vi "GeoData.vi"() -> ()   [LabVIEW 2017] (continued)
County\tH1\n39365\t28123\tUnion\tMS\tScott County\tH1\n39098\t28123\tLudlow\tMS\tScott County\tH1\n39117\t28123\tMorton\tMS\tScott County\tH1\n39152\t28123\tPulaski\tMS\tScott County\tH1\n39359\t28123\tSebastopol\tMS\tScott County\tH1\n39092\t28123\tLake\tMS\tScott County\tH1\n39145\t28123\tPelahatchie\tMS\tScott County\tH1\n39189\t28123\tWalnut grove\tMS\tScott County\tH1\n39074\t28123\tForest\tMS\tScott County\tH1\n39094\t28123\tLena\tMS\tScott County\tH1\n39057\t28123\tConehatta\tMS\tScott County\tH1\n39087\t28123\tHillsboro\tMS\tScott County\tH1\n39080\t28123\tHarperville\tMS\tScott County\tH1\n38721\t28125\tAnguilla\tMS\tSharkey County\tH1\n39159\t28125\tRolling fork\tMS\tSharkey County\tH1\n39054\t28125\tCary\tMS\tSharkey County\tH1\n39061\t28125\tDelta city\tMS\tSharkey County\tH1\n38765\t28125\tPanther burn\tMS\tSharkey County\tH1\n38748\t28125\tHollandale\tMS\tSharkey County\tH1\n39082\t28127\tHarrisville\tMS\tSimpson County\tH1\n39111\t28127\tMagee\tMS\tSimpson County\tH1\n39073\t28127\tFlorence\tMS\tSimpson County\tH1\n39119\t28127\tMount olive\tMS\tSimpson County\tH1\n39140\t28127\tNewhebron\tMS\tSimpson County\tH1\n39149\t28127\tPinola\tMS\tSimpson County\tH1\n39044\t28127\tBraxton\tMS\tSimpson County\tH1\n39114\t28127\tMendenhall\tMS\tSimpson County\tH1\n39062\t28127\tD lo\tMS\tSimpson County\tH1\n39116\t28129\tMize\tMS\tSmith County\tH1\n39042\t28129\tBrandon\tMS\tSmith County\tH1\n39111\t28129\tMagee\tMS\tSmith County\tH1\n39119\t28129\tMount olive\tMS\tSmith County\tH1\n39117\t28129\tMorton\tMS\tSmith County\tH1\n39152\t28129\tPulaski\tMS\tSmith County\tH1\n39153\t28129\tRaleigh\tMS\tSmith County\tH1\n39168\t28129\tTaylorsville\tMS\tSmith County\tH1\n39422\t28129\tBay springs\tMS\tSmith County\tH1\n39092\t28129\tLake\tMS\tSmith County\tH1\n39338\t28129\tLouin\tMS\tSmith County\tH1\n39074\t28129\tForest\tMS\tSmith County\tH1\n39114\t28129\tMendenhall\tMS\tSmith County\tH1\n39561\t28131\tMc henry\tMS\tStone County\tH1\n39456\t28131\tMc lain\tMS\tStone County\tH1\n39577\t28131\tWiggins\tMS\tStone County\tH1\n39574\t28131\tSaucier\tMS\tStone County\tH1\n39455\t28131\tLumberton\tMS\tStone County\tH1\n39452\t28131\tLucedale\tMS\tStone County\tH1\n39573\t28131\tPerkinston\tMS\tStone County\tH1\n38753\t28133\tInverness\tMS\tSunflower County\tH1\n38736\t28133\tDoddsville\tMS\tSunflower County\tH1\n38754\t28133\tIsola\tMS\tSunflower County\tH1\n38768\t28133\tRome\tMS\tSunflower County\tH1\n38751\t28133\tIndianola\tMS\tSunflower County\tH1\n38778\t28133\tSunflower\tMS\tSunflower County\tH1\n38761\t28133\tMoorhead\tMS\tSunflower County\tH1\n38756\t28133\tLeland\tMS\tSunflower County\tH1\n38759\t28133\tMerigold\tMS\tSunflower County\tH1\n39038\t28133\tBelzoni\tMS\tSunflower County\tH1\n38738\t28133\tParchman\tMS\tSunflower County\tH1\n38963\t28133\tTutwiler\tMS\tSunflower County\tH1\n38732\t28133\tCleveland\tMS\tSunflower County\tH1\n38737\t28133\tDrew\tMS\tSunflower County\tH1\n38773\t28133\tShaw\tMS\tSunflower County\tH1\n38771\t28133\tRuleville\tMS\tSunflower County\tH1\n38927\t28135\tEnid\tMS\tTallahatchie County\tH1\n38948\t28135\tOakland\tMS\tTallahatchie County\tH1\n38928\t28135\tGlendora\tMS\tTallahatchie County\tH1\n38920\t28135\tCascilla\tMS\tTallahatchie County\tH1\n38957\t28135\tSumner\tMS\tTallahatchie County\tH1\n38643\t28135\tLambert\tMS\tTallahatchie County\tH1\n38963\t28135\tTutwiler\tMS\tTallahatchie County\tH1\n38953\t28135\tScobey\tMS\tTallahatchie County\tH1\n38950\t28135\tPhilipp\tMS\tTallahatchie County\tH1\n38964\t28135\tVance\tMS\tTallahatchie County\tH1\n38966\t28135\tWebb\tMS\tTallahatchie County\tH1\n38901\t28135\tGrenada\tMS\tTallahatchie County\tH1\n38940\t28135\tHolcomb\tMS\tTallahatchie County\tH1\n38737\t28135\tDrew\tMS\tTallahatchie County\tH1\n38921\t28135\tCharleston\tMS\tTallahatchie County\tH1\n38961\t28135\tTillatoba\tMS\tTallahatchie County\tH1\n38962\t28135\tTippo\tMS\tTallahatchie County\tH1\n38635\t28137\tHolly springs\tMS\tTate County\tH1\n38619\t28137\tComo\tMS\tTate County\tH1\n38668\t28137\tSenatobia\tMS\tTate County\tH1\n38602\t28137\tArkabutla\tMS\tTate County\tH1\n38632\t28137\tHernando\tMS\tTate County\tH1\n38638\t28137\tIndependence\tMS\tTate County\tH1\n38618\t28137\tColdwater\tMS\tTate County\tH1\n38665\t28137\tSarah\tMS\tTate County\tH1\n38674\t28139\tTiplersville\tMS\tTippah County\tH1\n38603\t28139\tAshland\tMS\tTippah County\tH1\n38629\t28139\tFalkner\tMS\tTippah County\tH1\n38829\t28139\tBooneville\tMS\tTippah County\tH1\n38683\t28139\tWalnut\tMS\tTippah County\tH1\n38650\t28139\tMyrtle\tMS\tTippah County\tH1\n38610\t28139\tBlue mountain\tMS\tTippah County\tH1\n38625\t28139\tDumas\tMS\tTippah County\tH1\n38824\t28139\tBaldwyn\tMS\tTippah County\tH1\n38663\t28139\tRipley\tMS\tTippah County\tH1\n38852\t28141\tIuka\tMS\tTishomingo County\tH1\n38846\t28141\tGlen\tMS\tTishomingo County\tH1\n38873\t28141\tTishomingo\tMS\tTishomingo County\tH1\n38827\t28141\tBelmont\tMS\tTishomingo County\tH1\n38833\t28141\tBurnsville\tMS\tTishomingo County\tH1\n38847\t28141\tGolden\tMS\tTishomingo County\tH1\n38838\t28141\tDennis\tMS\tTishomingo County\tH1\n38626\t28143\tDundee\tMS\tTunica County\tH1\n38641\t28143\tLake cormorant\tMS\tTunica County\tH1\n38670\t28143\tSledge\tMS\tTunica County\tH1\n38621\t28143\tCrenshaw\tMS\tTunica County\tH1\n38665\t28143\tSarah\tMS\tTunica County\tH1\n38676\t28143\tTunica\tMS\tTunica County\tH1\n38664\t28143\tRobinsonville\tMS\tTunica County\tH1\n38849\t28145\tGuntown\tMS\tUnion County\tH1\n38652\t28145\tNew albany\tMS\tUnion County\tH1\n38828\t28145\tBlue springs\tMS\tUnion County\tH1\n38627\t28145\tEtta\tMS\tUnion County\tH1\n38841\t28145\tEcru\tMS\tUnion County\tH1\n38650\t28145\tMyrtle\tMS\tUnion County\tH1\n38610\t28145\tBlue mountain\tMS\tUnion County\tH1\n38625\t28145\tDumas\tMS\tUnion County\tH1\n38633\t28145\tHickory flat\tMS\tUnion County\tH1\n38824\t28145\tBaldwyn\tMS\tUnion County\tH1\n38663\t28145\tRipley\tMS\tUnion County\tH1\n38659\t28145\tPotts camp\tMS\tUnion County\tH1\n38871\t28145\tThaxton\tMS\tUnion County\tH1\n39652\t28147\tMagnolia\tMS\tWalthall County\tH1\n39667\t28147\tTylertown\tMS\tWalthall County\tH1\n39483\t28147\tFoxworth\tMS\tWalthall County\tH1\n39641\t28147\tJayess\tMS\tWalthall County\tH1\n39643\t28147\tKokomo\tMS\tWalthall County\tH1\n39478\t28147\tSandy hook\tMS\tWalthall County\tH1\n39648\t28147\tMccomb\tMS\tWalthall County\tH1\n39657\t28147\tOsyka\tMS\tWalthall County\tH1\n39181\t28149\tVicksburg\tMS\tWarren County\tH1\n39162\t28149\tSatartia\tMS\tWarren County\tH1\n39182\t28149\tVicksburg\tMS\tWarren County\tH1\n39183\t28149\tVicksburg\tMS\tWarren County\tH1\n39180\t28149\tVicksburg\tMS\tWarren County\tH1\n39156\t28149\tRedwood\tMS\tWarren County\tH1\n38721\t28151\tAnguilla\tMS\tWashington County\tH1\n38782\t28151\tWinterville\tMS\tWashington County\tH1\n38754\t28151\tIsola\tMS\tWashington County\tH1\n38751\t28151\tIndianola\tMS\tWashington County\tH1\n38744\t28151\tGlen allan\tMS\tWashington County\tH1\n38756\t28151\tLeland\tMS\tWashington County\tH1\n39038\t28151\tBelzoni\tMS\tWashington County\tH1\n38760\t28151\tMetcalfe\tMS\tWashington County\tH1\n38780\t28151\tWayside\tMS\tWashington County\tH1\n38723\t28151\tAvon\tMS\tWashington County\tH1\n38703\t28151\tGreenville\tMS\tWashington County\tH1\n38701\t28151\tGreenville\tMS\tWashington County\tH1\n38731\t28151\tChatham\tMS\tWashington County\tH1\n38773\t28151\tShaw\tMS\tWashington County\tH1\n38748\t28151\tHollandale\tMS\tWashington County\tH1\n38722\t28151\tArcola\tMS\tWashington County\tH1\n38776\t28151\tStoneville\tMS\tWashington County\tH1\n39443\t28153\tLaurel\tMS\tWayne County\tH1\n39360\t28153\tShubuta\tMS\tWayne County\tH1\n39367\t28153\tWaynesboro\tMS\tWayne County\tH1\n39362\t28153\tState line\tMS\tWayne County\tH1\n39476\t28153\tRichton\tMS\tWayne County\tH1\n39439\t28153\tHeidelberg\tMS\tWayne County\tH1\n39324\t28153\tClara\tMS\tWayne County\tH1\n39322\t28153\tBuckatunna\tMS\tWayne County\tH1\n39752\t28155\tMathiston\tMS\tWebster County\tH1\n39771\t28155\tWalthall\tMS\tWebster County\tH1\n38925\t28155\tDuck hill\tMS\tWebster County\tH1\n38929\t28155\tGore springs\tMS\tWebster County\tH1\n39744\t28155\tEupora\tMS\tWebster County\tH1\n39737\t28155\tBellefontaine\tMS\tWebster County\tH1\n39755\t28155\tPheba\tMS\tWebster County\tH1\n39767\t28155\tStewart\tMS\tWebster County\tH1\n38916\t28155\tCalhoun city\tMS\tWebster County\tH1\n39751\t28155\tMantee\tMS\tWebster County\tH1\n39750\t28155\tMaben\tMS\tWebster County\tH1\n39638\t28157\tGloster\tMS\tWilkinson County\tH1\n39633\t28157\tCrosby\tMS\tWilkinson County\tH1\n39631\t28157\tCentreville\tMS\tWilkinson County\tH1\n39669\t28157\tWoodville\tMS\tWilkinson County\tH1\n39350\t28159\tPhiladelphia\tMS\tWinston County\tH1\n39090\t28159\tKosciusko\tMS\tWinston County\tH1\n39339\t28159\tLouisville\tMS\tWinston County\tH1\n39772\t28159\tWeir\tMS\tWinston County\tH1\n39108\t28159\tMc cool\tMS\tWinston County\tH1\n39354\t28159\tPreston\tMS\tWinston County\tH1\n39346\t28159\tNoxapater\tMS\tWinston County\tH1\n39735\t28159\tAckerman\tMS\tWinston County\tH1\n39769\t28159\tSturgis\tMS\tWinston County\tH1\n39341\t28159\tMacon\tMS\tWinston County\tH1\n38927\t28161\tEnid\tMS\tYalobusha County\tH1\n38948\t28161\tOakland\tMS\tYalobusha County\tH1\n38922\t28161\tCoffeeville\tMS\tYalobusha County\tH1\n38953\t28161\tScobey\tMS\tYalobusha County\tH1\n38965\t28161\tWater valley\tMS\tYalobusha County\tH1\n38961\t28161\tTillatoba\tMS\tYalobusha County\tH1\n39162\t28163\tSatartia\tMS\tYazoo County\tH1\n39194\t28163\tYazoo city\tMS\tYazoo County\tH1\n39159\t28163\tRolling fork\tMS\tYazoo County\tH1\n39040\t28163\tBentonia\tMS\tYazoo County\tH1\n39146\t28163\tPickens\tMS\tYazoo County\tH1\n39166\t28163\tSilver city\tMS\tYazoo County\tH1\n39088\t28163\tHolly bluff\tMS\tYazoo County\tH1\n39173\t28163\tTinsley\tMS\tYazoo County\tH1\n39095\t28163\tLexington\tMS\tYazoo County\tH1\n39039\t28163\tBenton\tMS\tYazoo County\tH1\n39179\t28163\tVaughan\tMS\tYazoo County\tH1\n39097\t28163\tLouise\tMS\tYazoo County\tH1\n63501\t29001\tKirksville\tMO\tAdair County\tH1\n63540\t29001\tGibbs\tMO\tAdair County\tH1\n63547\t29001\tHurdland\tMO\tAdair County\tH1\n63559\t29001\tNovinger\tMO\tAdair County\tH1\n63557\t29001\tNew boston\tMO\tAdair County\tH1\n63549\t29001\tLa plata\tMO\tAdair County\tH1\n63544\t29001\tGreen castle\tMO\tAdair County\tH1\n63546\t29001\tGreentop\tMO\tAdair County\tH1\n63533\t29001\tBrashear\tMO\tAdair County\tH1\n64455\t29003\tGraham\tMO\tAndrew County\tH1\n64485\t29003\tSavannah\tMO\tAndrew County\tH1\n64421\t29003\tAmazonia\tMO\tAndrew County\tH1\n64449\t29003\tFillmore\tMO\tAndrew County\tH1\n64480\t29003\tRea\tMO\tAndrew County\tH1\n64463\t29003\tKing city\tMO\tAndrew County\tH1\n64430\t29003\tClarksdale\tMO\tAndrew County\tH1\n64436\t29003\tCosby\tMO\tAndrew County\tH1\n64423\t29003\tBarnard\tMO\tAndrew County\tH1\n64459\t29003\tHelena\tMO\tAndrew County\tH1\n64427\t29003\tBolckow\tMO\tAndrew County\tH1\n64483\t29003\tRosendale\tMO\tAndrew County\tH1\n64505\t29003\tSaint joseph\tMO\tAndrew County\tH1\n64457\t29003\tGuilford\tMO\tAndrew County\tH1\n64494\t29003\tUnion star\tMO\tAndrew County\tH1\n64507\t29003\tSaint joseph\tMO\tAndrew County\tH1\n64506\t29003\tSaint joseph\tMO\tAndrew County\tH1\n64491\t29005\tTarkio\tMO\tAtchison County\tH1\n64437\t29005\tCraig\tMO\tAtchison County\tH1\n64496\t29005\tWatson\tMO\tAtchison County\tH1\n64498\t29005\tWestboro\tMO\tAtchison County\tH1\n64428\t29005\tBurlington junction\tMO\tAtchison County\tH1\n64446\t29005\tFairfax\tMO\tAtchison County\tH1\n64487\t29005\tSkidmore\tMO\tAtchison County\tH1\n64482\t29005\tRock port\tMO\tAtchison County\tH1\n65231\t29007\tAuxvasse\tMO\tAudrain County\tH1\n65265\t29007\tMexico\tMO\tAudrain County\tH1\n65280\t29007\tRush hill\tMO\tAudrain County\tH1\n63345\t29007\tFarber\tMO\tAudrain County\tH1\n65240\t29007\tCentralia\tMO\tAudrain County\tH1\n65285\t29007\tThompson\tMO\tAudrain County\tH1\n63384\t29007\tWellsville\tMO\tAudrain County\tH1\n65284\t29007\tSturgeon\tMO\tAudrain County\tH1\n63382\t29007\tVandalia\tMO\tAudrain County\tH1\n63352\t29007\tLaddonia\tMO\tAudrain County\tH1\n63359\t29007\tMiddletown\tMO\tAudrain County\tH1\n65232\t29007\tBenton city\tMO\tAudrain County\tH1\n65243\t29007\tClark\tMO\tAudrain County\tH1\n65264\t29007\tMartinsburg\tMO\tAudrain County\tH1\n65656\t29009\tGalena\tMO\tBarry County\tH1\n65633\t29009\tCrane\tMO\tBarry County\tH1\n65625\t29009\tCassville\tMO\tBarry County\tH1\n65654\t29009\tFreistatt\tMO\tBarry County\tH1\n65647\t29009\tExeter\tMO\tBarry County\tH1\n65658\t29009\tGolden\tMO\tBarry County\tH1\n65641\t29009\tEagle rock\tMO\tBarry County\tH1\n64874\t29009\tWheaton\tMO\tBarry County\tH1\n65623\t29009\tButterfield\tMO\tBarry County\tH1\n65605\t29009\tAurora\tMO\tBarry County\tH1\n65723\t29009\tPierce city\tMO\tBarry County\tH1\n65708\t29009\tMonett\tMO\tBarry County\tH1\n65769\t29009\tVerona\tMO\tBarry County\tH1\n65747\t29009\tShell knob\tMO\tBarry County\tH1\n65772\t29009\tWashburn\tMO\tBarry County\tH1\n64842\t29009\tFairview\tMO\tBarry County\tH1\n65745\t29009\tSeligman\tMO\tBarry County\tH1\n65734\t29009\tPurdy\tMO\tBarry County\tH1\n64855\t29011\tOronogo\tMO\tBarton County\tH1\n64762\t29011\tLiberal\tMO\tBarton County\tH1\n64832\t29011\tAsbury\tMO\tBarton County\tH1\n64728\t29011\tBronaugh\tMO\tBarton County\tH1\n64748\t29011\tGolden city\tMO\tBarton County\tH1\n64759\t29011\tLamar\tMO\tBarton County\tH1\n64784\t29011\tSheldon\tMO\tBarton County\tH1\n64769\t29011\tMindenmines\tMO\tBarton County\tH1\n64755\t29011\tJasper\tMO\tBarton County\tH1\n64780\t29013\tRockville\tMO\tBates County\tH1\n64720\t29013\tAdrian\tMO\tBates County\tH1\n64647\t29013\tJameson\tMO\tBates County\tH1\n64730\t29013\tButler\tMO\tBates County\tH1\n64724\t29013\tAppleton city\tMO\tBates County\tH1\n64745\t29013\tFoster\tMO\tBates County\tH1\n64752\t29013\tHume\tMO\tBates County\tH1\n64779\t29013\tRich hill\tMO\tBates County\tH1\n64742\t29013\tDrexel\tMO\tBates County\tH1\n64722\t29013\tAmoret\tMO\tBates County\tH1\n64788\t29013\tUrich\tMO\tBates County\tH1\n64723\t29013\tAmsterdam\tMO\tBates County\tH1\n65338\t29015\tLincoln\tMO\tBenton County\tH1\n65634\t29015\tCross timbers\tMO\tBenton County\tH1\n64735\t29015\tClinton\tMO\tBenton County\tH1\n64776\t29015\tOsceola\tMO\tBenton County\tH1\n65326\t29015\tEdwards\tMO\tBenton County\tH1\n65324\t29015\tClimax springs\tMO\tBenton County\tH1\n65325\t29015\tCole camp\tMO\tBenton County\tH1\n65355\t29015\tWarsaw\tMO\tBenton County\tH1\n65360\t29015\tWindsor\tMO\tBenton County\tH1\n65779\t29015\tWheatland\tMO\tBenton County\tH1\n65735\t29015\tQuincy\tMO\tBenton County\tH1\n65345\t29015\tMora\tMO\tBenton County\tH1\n65335\t29015\tIonia\tMO\tBenton County\tH1\n63787\t29017\tZalma\tMO\tBollinger County\tH1\n63782\t29017\tSturdivant\tMO\tBollinger County\tH1\n63730\t29017\tAdvance\tMO\tBollinger County\tH1\n63662\t29017\tPatton\tMO\tBollinger County\tH1\n63750\t29017\tGipsy\tMO\tBollinger County\tH1\n63760\t29017\tLeopold\tMO\tBollinger County\tH1\n63751\t29017\tGlenallen\tMO\tBollinger County\tH1\n63764\t29017\tMarble hill\tMO\tBollinger County\tH1\n63781\t29017\tSedgewickville\tMO\tBollinger County\tH1\n65202\t29019\tColumbia\tMO\tBoone County\tH1\n65201\t29019\tColumbia\tMO\tBoone County\tH1\n65279\t29019\tRocheport\tMO\tBoone County\tH1\n65010\t29019\tAshland\tMO\tBoone County\tH1\n65205\t29019\tColumbia\tMO\tBoone County\tH1\n65256\t29019\tHarrisburg\tMO\tBoone County\tH1\n65216\t29019\tColumbia\tMO\tBoone County\tH1\n65039\t29019\tHartsburg\tMO\tBoone County\tH1\n65240\t29019\tCentralia\tMO\tBoone County\tH1\n65255\t29019\tHallsville\tMO\tBoone County\tH1\n65284\t29019\tSturgeon\tMO\tBoone County\tH1\n65217\t29019\tColumbia\tMO\tBoone County\tH1\n65218\t29019\tColumbia\tMO\tBoone County\tH1\n65212\t29019\tColumbia\tMO\tBoone County\tH1\n65215\t29019\tColumbia\tMO\tBoone County\tH1\n65203\t29019\tColumbia\tMO\tBoone County\tH1\n65211\t29019\tColumbia\tMO\tBoone County\tH1\n65243\t29019\tClark\tMO\tBoone County\tH1\n65299\t29019\tColumbia\tMO\tBoone County\tH1\n64439\t29021\tDearborn\tMO\tBuchanan County\tH1\n64490\t29021\tStewartsville\tMO\tBuchanan County\tH1\n64504\t29021\tSaint joseph\tMO\tBuchanan County\tH1\n64443\t29021\tEaston\tMO\tBuchanan County\tH1\n64444\t29021\tEdgerton\tMO\tBuchanan County\tH1\n64502\t29021\tSaint joseph\tMO\tBuchanan County\tH1\n64440\t29021\tDe kalb\tMO\tBuchanan County\tH1\n64454\t29021\tGower\tMO\tBuchanan County\tH1\n64430\t29021\tClarksdale\tMO\tBuchanan County\tH1\n64436\t29021\tCosby\tMO\tBuchanan County\tH1\n64448\t29021\tFaucett\tMO\tBuchanan County\tH1\n64508\t29021\tSaint joseph\tMO\tBuchanan County\tH1\n64401\t29021\tAgency\tMO\tBuchanan County\tH1\n64503\t29021\tSaint joseph\tMO\tBuchanan County\tH1\n64484\t29021\tRushville\tMO\tBuchanan County\tH1\n64501\t29021\tSaint joseph\tMO\tBuchanan County\tH1\n64505\t29021\tSaint joseph\tMO\tBuchanan County\tH1\n64507\t29021\tSaint joseph\tMO\tBuchanan County\tH1\n64506\t29021\tSaint joseph\tMO\tBuchanan County\tH1\n63962\t29023\tRombauer\tMO\tButler County\tH1\n63954\t29023\tNeelyville\tMO\tButler County\tH1\n63901\t29023\tPoplar bluff\tMO\tButler County\tH1\n63932\t29023\tBroseley\tMO\tButler County\tH1\n63937\t29023\tEllsinore\tMO\tButler County\tH1\n63966\t29023\tWappapello\tMO\tButler County\tH1\n63945\t29023\tHarviell\tMO\tButler County\tH1\n63967\t29023\tWilliamsville\tMO\tButler County\tH1\n63961\t29023\tQulin\tMO\tButler County\tH1\n63940\t29023\tFisk\tMO\tButler County\tH1\n63902\t29023\tPoplar bluff\tMO\tButler County\tH1\n64465\t29025\tLathrop\tMO\tCaldwell County\tH1\n64671\t29025\tPolo\tMO\tCaldwell County\tH1\n64644\t29025\tHamilton\tMO\tCaldwell County\tH1\n64650\t29025\tKingston\tMO\tCaldwell County\tH1\n64625\t29025\tBreckenridge\tMO\tCaldwell County\tH1\n64637\t29025\tCowgill\tMO\tCaldwell County\tH1\n64062\t29025\tLawson\tMO\tCaldwell County\tH1\n64649\t29025\tKidder\tMO\tCaldwell County\tH1\n64624\t29025\tBraymer\tMO\tCaldwell County\tH1\n64429\t29025\tCameron\tMO\tCaldwell County\tH1\n65202\t29027\tColumbia\tMO\tCallaway County\tH1\n65069\t29027\tRhineland\tMO\tCallaway County\tH1\n65201\t29027\tColumbia\tMO\tCallaway County\tH1\n63388\t29027\tWilliamsburg\tMO\tCallaway County\tH1\n65059\t29027\tMokane\tMO\tCallaway County\tH1\n65231\t29027\tAuxvasse\tMO\tCallaway County\tH1\n65265\t29027\tMexico\tMO\tCallaway County\tH1\n65067\t29027\tPortland\tMO\tCallaway County\tH1\n65039\t29027\tHartsburg\tMO\tCallaway County\tH1\n65240\t29027\tCentralia\tMO\tCallaway County\tH1\n65251\t29027\tFulton\tMO\tCallaway County\tH1\n65101\t29027\tJefferson city\tMO\tCallaway County\tH1\n63384\t29027\tWellsville\tMO\tCallaway County\tH1\n65077\t29027\tSteedman\tMO\tCallaway County\tH1\n65262\t29027\tKingdom city\tMO\tCallaway County\tH1\n65043\t29027\tHolts summit\tMO\tCallaway County\tH1\n65063\t29027\tNew bloomfield\tMO\tCallaway County\tH1\n65080\t29027\tTebbetts\tMO\tCallaway County\tH1\n63361\t29027\tMontgomery city\tMO\tCallaway County\tH1\n65264\t29027\tMartinsburg\tMO\tCallaway County\tH1\n65536\t29029\tLebanon\tMO\tCamden County\tH1\n65452\t29029\tCrocker\tMO\tCamden County\tH1\n65065\t29029\tOsage beach\tMO\tCamden County\tH1\n65037\t29029\tGravois mills\tMO\tCamden County\tH1\n65047\t29029\tKaiser\tMO\tCamden County\tH1\n65634\t29029\tCross timbers\tMO\tCamden County\tH1\n65787\t29029\tRoach\tMO\tCamden County\tH1\n65017\t29029\tBrumley\tMO\tCamden County\tH1\n65567\t29029\tStoutland\tMO\tCamden County\tH1\n65556\t29029\tRichland\tMO\tCamden County\tH1\n65079\t29029\tSunrise beach\tMO\tCamden County\tH1\n65326\t29029\tEdwards\tMO\tCamden County\tH1\n65591\t29029\tMontreal\tMO\tCamden County\tH1\n65324\t29029\tClimax springs\tMO\tCamden County\tH1\n65786\t29029\tMacks creek\tMO\tCamden County\tH1\n65020\t29029\tCamdenton\tMO\tCamden County\tH1\n65049\t29029\tLake ozark\tMO\tCamden County\tH1\n65052\t29029\tLinn creek\tMO\tCamden County\tH1\n63732\t29031\tAltenburg\tMO\tCape Girardeau County\tH1\n63730\t29031\tAdvance\tMO\tCape Girardeau County\tH1\n63785\t29031\tWhitewater\tMO\tCape Girardeau County\tH1\n63755\t29031\tJackson\tMO\tCape Girardeau County\tH1\n63771\t29031\tOran\tMO\tCape Girardeau County\tH1\n63752\t29031\tGordonville\tMO\tCape Girardeau County\tH1\n63740\t29031\tChaffee\tMO\tCape Girardeau County\tH1\n63780\t29031\tScott city\tMO\tCape Girardeau County\tH1\n63769\t29031\tOak ridge\tMO\tCape Girardeau County\tH1\n63770\t29031\tOld appleton\tMO\tCape Girardeau County\tH1\n63703\t29031\tCape girardeau\tMO\tCape Girardeau County\tH1\n63775\t29031\tPerryville\tMO\tCape Girardeau County\tH1\n63766\t29031\tMillersville\tMO\tCape Girardeau County\tH1\n63739\t29031\tBurfordville\tMO\tCape Girardeau County\tH1\n63743\t29031\tDaisy\tMO\tCape Girardeau County\tH1\n63745\t29031\tDutchtown\tMO\tCape Girardeau County\tH1\n63779\t29031\tPocahontas\tMO\tCape Girardeau County\tH1\n63747\t29031\tFriedheim\tMO\tCape Girardeau County\tH1\n63701\t29031\tCape girardeau\tMO\tCape Girardeau County\tH1\n63764\t29031\tMarble hill\tMO\tCape Girardeau County\tH1\n63702\t29031\tCape girardeau\tMO\tCape Girardeau County\tH1\n63744\t29031\tDelta\tMO\tCape Girardeau County\tH1\n64643\t29033\tHale\tMO\tCarroll County\tH1\n64622\t29033\tBogard\tMO\tCarroll County\tH1\n64680\t29033\tStet\tMO\tCarroll County\tH1\n64639\t29033\tDe witt\tMO\tCarroll County\tH1\n64035\t29033\tHardin\tMO\tCarroll County\tH1\n64638\t29033\tDawn\tMO\tCarroll County\tH1\n64633\t29033\tCarrollton\tMO\tCarroll County\tH1\n64624\t29033\tBraymer\tMO\tCarroll County\tH1\n64623\t29033\tBosworth\tMO\tCarroll County\tH1\n64668\t29033\tNorborne\tMO\tCarroll County\tH1\n64682\t29033\tTina\tMO\tCarroll County\tH1\n63965\t29035\tVan buren\tMO\tCarter County\tH1\n63901\t29035\tPoplar bluff\tMO\tCarter County\tH1\n63937\t29035\tEllsinore\tMO\tCarter County\tH1\n63943\t29035\tGrandin\tMO\tCarter County\tH1\n63941\t29035\tFremont\tMO\tCarter County\tH1\n64078\t29037\tPeculiar\tMO\tCass County\tH1\n64725\t29037\tArchie\tMO\tCass County\tH1\n64746\t29037\tFreeman\tMO\tCass County\tH1\n64034\t29037\tGreenwood\tMO\tCass County\tH1\n64701\t29037\tHarrisonville\tMO\tCass County\tH1\n64080\t29037\tPleasant hill\tMO\tCass County\tH1\n64720\t29037\tAdrian\tMO\tCass County\tH1\n64083\t29037\tRaymore\tMO\tCass County\tH1\n64090\t29037\tStrasburg\tMO\tCass County\tH1\n64743\t29037\tEast lynne\tMO\tCass County\tH1\n64070\t29037\tLone jack\tMO\tCass County\tH1\n64061\t29037\tKingsville\tMO\tCass County\tH1\n64747\t29037\tGarden city\tMO\tCass County\tH1\n64742\t29037\tDrexel\tMO\tCass County\tH1\n64147\t29037\tKansas city\tMO\tCass County\tH1\n64734\t29037\tCleveland\tMO\tCass County\tH1\n64012\t29037\tBelton\tMO\tCass County\tH1\n64040\t29037\tHolden\tMO\tCass County\tH1\n64082\t29037\tLees summit\tMO\tCass County\tH1\n64739\t29037\tCreighton\tMO\tCass County\tH1\n65601\t29039\tAldrich\tMO\tCedar County\tH1\n65785\t29039\tStockton\tMO\tCedar County\tH1\n65674\t29039\tHumansville\tMO\tCedar County\tH1\n65649\t29039\tFair play\tMO\tCedar County\tH1\n65635\t29039\tDadeville\tMO\tCedar County\tH1\n64744\t29039\tEl dorado springs\tMO\tCedar County\tH1\n64756\t29039\tJerico springs\tMO\tCedar County\tH1\n65640\t29039\tDunnegan\tMO\tCedar County\tH1\n64784\t29039\tSheldon\tMO\tCedar County\tH1\n65607\t29039\tCaplinger mills\tMO\tCedar County\tH1\n64676\t29041\tRothville\tMO\tChariton County\tH1\n65244\t29041\tClifton hill\tMO\tChariton County\tH1\n65281\t29041\tSalisbury\tMO\tChariton County\tH1\n64658\t29041\tMarceline\tMO\tChariton County\tH1\n65254\t29041\tGlasgow\tMO\tChariton County\tH1\n65246\t29041\tDalton\tMO\tChariton County\tH1\n64628\t29041\tBrookfield\tMO\tChariton County\tH1\n65261\t29041\tKeytesville\tMO\tChariton County\tH1\n63558\t29041\tNew cambria\tMO\tChariton County\tH1\n65236\t29041\tBrunswick\tMO\tChariton County\tH1\n65286\t29041\tTriplett\tMO\tChariton County\tH1\n64660\t29041\tMendon\tMO\tChariton County\tH1\n64681\t29041\tSumner\tMO\tChariton County\tH1\n65714\t29043\tNixa\tMO\tChristian County\tH1\n65656\t29043\tGalena\tMO\tChristian County\tH1\n65614\t29043\tBradleyville\tMO\tChristian County\tH1\n65720\t29043\tOldfield\tMO\tChristian County\tH1\n65705\t29043\tMarionville\tMO\tChristian County\tH1\n65669\t29043\tHighlandville\tMO\tChristian County\tH1\n65728\t29043\tPonce de leon\tMO\tChristian County\tH1\n65721\t29043\tOzark\tMO\tChristian County\tH1\n65759\t29043\tTaneyville\tMO\tChristian County\tH1\n65771\t29043\tWalnut shade\tMO\tChristian County\tH1\n65610\t29043\tBillings\tMO\tChristian County\tH1\n65738\t29043\tRepublic\tMO\tChristian County\tH1\n65620\t29043\tBruner\tMO\tChristian County\tH1\n65619\t29043\tBrookline\tMO\tChristian County\tH1\n65653\t29043\tForsyth\tMO\tChristian County\tH1\n65737\t29043\tReeds spring\tMO\tChristian County\tH1\n65652\t29043\tFordland\tMO\tChristian County\tH1\n65631\t29043\tClever\tMO\tChristian County\tH1\n65754\t29043\tSpokane\tMO\tChristian County\tH1\n65753\t29043\tSparta\tMO\tChristian County\tH1\n65742\t29043\tRogersville\tMO\tChristian County\tH1\n65629\t29043\tChadwick\tMO\tChristian County\tH1\n65657\t29043\tGarrison\tMO\tChristian County\tH1\n65630\t29043\tChestnutridge\tMO\tChristian County\tH1\n63445\t29045\tKahoka\tMO\tClark County\tH1\n63453\t29045\tLuray\tMO\tClark County\tH1\n63465\t29045\tRevere\tMO\tClark County\tH1\n63435\t29045\tCanton\tMO\tClark County\tH1\n63430\t29045\tAlexandria\tMO\tClark County\tH1\n63472\t29045\tWayland\tMO\tClark County\tH1\n63466\t29045\tSaint patrick\tMO\tClark County\tH1\n63474\t29045\tWyaconda\tMO\tClark County\tH1\n63432\t29045\tArbela\tMO\tClark County\tH1\n64116\t29047\tKansas city\tMO\tClay County\tH1\n64161\t29047\tKansas city\tMO\tClay County\tH1\n64165\t29047\tKansas city\tMO\tClay County\tH1\n64118\t29047\tKansas city\tMO\tClay County\tH1\n64150\t29047\tRiverside\tMO\tClay County\tH1\n64024\t29047\tExcelsior springs\tMO\tClay County\tH1\n64131\t29047\tKansas city\tMO\tClay County\tH1\n64151\t29047\tKansas city\tMO\tClay County\tH1\n64072\t29047\tMissouri city\tMO\tClay County\tH1\n64144\t29047\tKansas city\tMO\tClay County\tH1\n64089\t29047\tSmithville\tMO\tClay County\tH1\n64077\t29047\tOrrick\tMO\tClay County\tH1\n64158\t29047\tKansas city\tMO\tClay County\tH1\n64163\t29047\tKansas city\tMO\tClay County\tH1\n64166\t29047\tKansas city\tMO\tClay County\tH1\n64188\t29047\tKansas city\tMO\tClay County\tH1\n64069\t29047\tLiberty\tMO\tClay County\tH1\n64068\t29047\tLiberty\tMO\tClay County\tH1\n64062\t29047\tLawson\tMO\tClay County\tH1\n64157\t29047\tKansas city\tMO\tClay County\tH1\n64073\t29047\tMosby\tMO\tClay County\tH1\n64114\t29047\tKansas city\tMO\tClay County\tH1\n64060\t29047\tKearney\tMO\tClay County\tH1\n64119\t29047\tKansas city\tMO\tClay County\tH1\n64156\t29047\tKansas city\tMO\tClay County\tH1\n64117\t29047\tKansas city\tMO\tClay County\tH1\n64048\t29047\tHolt\tMO\tClay County\tH1\n64155\t29047\tKansas city\tMO\tClay County\tH1\n64167\t29047\tKansas city\tMO\tClay County\tH1\n64492\t29047\tTrimble\tMO\tClay County\tH1\n64162\t29047\tKansas city\tMO\tClay County\tH1\n64465\t29049\tLathrop\tMO\tClinton County\tH1\n64490\t29049\tStewartsville\tMO\tClinton County\tH1\n64493\t29049\tTurney\tMO\tClinton County\tH1\n64474\t29049\tOsborn\tMO\tClinton County\tH1\n64089\t29049\tSmithville\tMO\tClinton County\tH1\n64444\t29049\tEdgerton\tMO\tClinton County\tH1\n64062\t29049\tLawson\tMO\tClinton County\tH1\n64454\t29049\tGower\tMO\tClinton County\tH1\n64429\t29049\tCameron\tMO\tClinton County\tH1\n64477\t29049\tPlattsburg\tMO\tClinton County\tH1\n64048\t29049\tHolt\tMO\tClinton County\tH1\n64492\t29049\tTrimble\tMO\tClinton County\tH1\n65105\t29051\tJefferson city\tMO\tCole County\tH1\n65032\t29051\tEugene\tMO\tCole County\tH1\n65058\t29051\tMeta\tMO\tCole County\tH1\n65101\t29051\tJefferson city\tMO\tCole County\tH1\n65076\t29051\tSaint thomas\tMO\tCole County\tH1\n65110\t29051\tJefferson city\tMO\tCole County\tH1\n65102\t29051\tJefferson city\tMO\tCole County\tH1\n65104\t29051\tJefferson city\tMO\tCole County\tH1\n65023\t29051\tCentertown\tMO\tCole County\tH1\n65040\t29051\tHenley\tMO\tCole County\tH1\n65053\t29051\tLohman\tMO\tCole County\tH1\n65074\t29051\tRussellville\tMO\tCole County\tH1\n65103\t29051\tJefferson city\tMO\tCole County\tH1\n65111\t29051\tJefferson city\tMO\tCole County\tH1\n65046\t29051\tJamestown\tMO\tCole County\tH1\n65109\t29051\tJefferson city\tMO\tCole County\tH1\n65233\t29053\tBoonville\tMO\tCooper County\tH1\n65287\t29053\tWooldridge\tMO\tCooper County\tH1\n65237\t29053\tBunceton\tMO\tCooper County\tH1\n65081\t29053\tTipton\tMO\tCooper County\tH1\n65350\t29053\tSmithton\tMO\tCooper County\tH1\n65018\t29053\tCalifornia\tMO\tCooper County\tH1\n65322\t29053\tBlackwater\tMO\tCooper County\tH1\n65347\t29053\tNelson\tMO\tCooper County\tH1\n65301\t29053\tSedalia\tMO\tCooper County\tH1\n65025\t29053\tClarksburg\tMO\tCooper County\tH1\n65276\t29053\tPilot grove\tMO\tCooper County\tH1\n65068\t29053\tPrairie home\tMO\tCooper County\tH1\n65046\t29053\tJamestown\tMO\tCooper County\tH1\n65348\t29053\tOtterville\tMO\tCooper County\tH1\n65354\t29053\tSyracuse\tMO\tCooper County\tH1\n65559\t29055\tSaint james\tMO\tCrawford County\tH1\n65441\t29055\tBourbon\tMO\tCrawford County\tH1\n65586\t29055\tWesco\tMO\tCrawford County\tH1\n65456\t29055\tDavisville\tMO\tCrawford County\tH1\n63080\t29055\tSullivan\tMO\tCrawford County\tH1\n65565\t29055\tSteelville\tMO\tCrawford County\tH1\n65560\t29055\tSalem\tMO\tCrawford County\tH1\n65453\t29055\tCuba\tMO\tCrawford County\tH1\n65066\t29055\tOwensville\tMO\tCrawford County\tH1\n65449\t29055\tCook sta\tMO\tCrawford County\tH1\n65535\t29055\tLeasburg\tMO\tCrawford County\tH1\n65566\t29055\tViburnum\tMO\tCrawford County\tH1\n65446\t29055\tCherryville\tMO\tCrawford County\tH1\n65601\t29057\tAldrich\tMO\tDade County\tH1\n65682\t29057\tLockwood\tMO\tDade County\tH1\n65785\t29057\tStockton\tMO\tDade County\tH1\n65752\t29057\tSouth greenfield\tMO\tDade County\tH1\n65770\t29057\tWalnut grove\tMO\tDade County\tH1\n65603\t29057\tArcola\tMO\tDade County\tH1\n65604\t29057\tAsh grove\tMO\tDade County\tH1\n65635\t29057\tDadeville\tMO\tDade County\tH1\n65646\t29057\tEverton\tMO\tDade County\tH1\n65661\t29057\tGreenfield\tMO\tDade County\tH1\n64748\t29057\tGolden city\tMO\tDade County\tH1\n64759\t29057\tLamar\tMO\tDade County\tH1\n64756\t29057\tJerico springs\tMO\tDade County\tH1\n65536\t29059\tLebanon\tMO\tDallas County\tH1\n65622\t29059\tBuffalo\tMO\tDallas County\tH1\n65632\t29059\tConway\tMO\tDallas County\tH1\n65732\t29059\tPreston\tMO\tDallas County\tH1\n65722\t29059\tPhillipsburg\tMO\tDallas County\tH1\n65463\t29059\tEldridge\tMO\tDallas County\tH1\n65644\t29059\tElkland\tMO\tDallas County\tH1\n65590\t29059\tLong lane\tMO\tDallas County\tH1\n65783\t29059\tWindyville\tMO\tDallas County\tH1\n65648\t29059\tFair grove\tMO\tDallas County\tH1\n65786\t29059\tMacks creek\tMO\tDallas County\tH1\n65767\t29059\tUrbana\tMO\tDallas County\tH1\n65685\t29059\tLouisburg\tMO\tDallas County\tH1\n65764\t29059\tTunas\tMO\tDallas County\tH1\n64689\t29061\tWinston\tMO\tDaviess County\tH1\n64640\t29061\tGallatin\tMO\tDaviess County\tH1\n64620\t29061\tAltamont\tMO\tDaviess County\tH1\n64644\t29061\tHamilton\tMO\tDaviess County\tH1\n64647\t29061\tJameson\tMO\tDaviess County\tH1\n64497\t29061\tWeatherby\tMO\tDaviess County\tH1\n64625\t29061\tBreckenridge\tMO\tDaviess County\tH1\n64670\t29061\tPattonsburg\tMO\tDaviess County\tH1\n64649\t29061\tKidder\tMO\tDaviess County\tH1\n64601\t29061\tChillicothe\tMO\tDaviess County\tH1\n64648\t29061\tJamesport\tMO\tDaviess County\tH1\n64642\t29061\tGilman city\tMO\tDaviess County\tH1\n64429\t29061\tCameron\tMO\tDaviess County\tH1\n64657\t29061\tMc fall\tMO\tDaviess County\tH1\n64683\t29061\tTrenton\tMO\tDaviess County\tH1\n64636\t29061\tCoffey\tMO\tDaviess County\tH1\n64654\t29061\tLock springs\tMO\tDaviess County\tH1\n64422\t29063\tAmity\tMO\tDeKalb County\tH1\n64490\t29063\tStewartsville\tMO\tDeKalb County\tH1\n64474\t29063\tOsborn\tMO\tDeKalb County\tH1\n64497\t29063\tWeatherby\tMO\tDeKalb County\tH1\n64463\t29063\tKing city\tMO\tDeKalb County\tH1\n64430\t29063\tClarksdale\tMO\tDeKalb County\tH1\n64670\t29063\tPattonsburg\tMO\tDeKalb County\tH1\n64469\t29063\tMaysville\tMO\tDeKalb County\tH1\n64429\t29063\tCameron\tMO\tDeKalb County\tH1\n64494\t29063\tUnion star\tMO\tDeKalb County\tH1\n63638\t29065\tEllington\tMO\tDent County\tH1\n63629\t29065\tBunker\tMO\tDent County\tH1\n65541\t29065\tLenox\tMO\tDent County\tH1\n65401\t29065\tRolla\tMO\tDent County\tH1\n65462\t29065\tEdgar springs\tMO\tDent County\tH1\n65501\t29065\tJadwin\tMO\tDent County\tH1\n65532\t29065\tLake spring\tMO\tDent County\tH1\n65560\t29065\tSalem\tMO\tDent County\tH1\n65542\t29065\tLicking\tMO\tDent County\tH1\n65440\t29065\tBoss\tMO\tDent County\tH1\n65720\t29067\tOldfield\tMO\tDouglas County\tH1\n65638\t29067\tDrury\tMO\tDouglas County\tH1\n65775\t29067\tWest plains\tMO\tDouglas County\tH1\n65608\t29067\tAva\tMO\tDouglas County\tH1\n65652\t29067\tFordland\tMO\tDouglas County\tH1\n65755\t29067\tSquires\tMO\tDouglas County\tH1\n65768\t29067\tVanzant\tMO\tDouglas County\tH1\n65715\t29067\tNoble\tMO\tDouglas County\tH1\n63857\t29069\tKennett\tMO\tDunklin County\tH1\n63863\t29069\tMalden\tMO\tDunklin County\tH1\n63877\t29069\tSteele\tMO\tDunklin County\tH1\n63822\t29069\tBernie\tMO\tDunklin County\tH1\n63875\t29069\tRives\tMO\tDunklin County\tH1\n63933\t29069\tCampbell\tMO\tDunklin County\tH1\n63829\t29069\tCardwell\tMO\tDunklin County\tH1\n63876\t29069\tSenath\tMO\tDunklin County\tH1\n63880\t29069\tWhiteoak\tMO\tDunklin County\tH1\n63821\t29069\tArbyrd\tMO\tDunklin County\tH1\n63837\t29069\tClarkton\tMO\tDunklin County\tH1\n63855\t29069\tHornersville\tMO\tDunklin County\tH1\n63847\t29069\tGibson\tMO\tDunklin County\tH1\n63849\t29069\tGobler\tMO\tDunklin County\tH1\n63852\t29069\tHolcomb\tMO\tDunklin County\tH1\n63055\t29071\tLabadie\tMO\tFranklin County\tH1\n63039\t29071\tGray summit\tMO\tFranklin County\tH1\n63061\t29071\tLuebbering\tMO\tFranklin County\tH1\n63084\t29071\tUnion\tMO\tFranklin County\tH1\n63089\t29071\tVilla ridge\tMO\tFranklin County\tH1\n65441\t29071\tBourbon\tMO\tFranklin County\tH1\n63005\t29071\tChesterfield\tMO\tFranklin County\tH1\n63079\t29071\tStanton\tMO\tFranklin County\tH1\n63056\t29071\tLeslie\tMO\tFranklin County\tH1\n63068\t29071\tNew haven\tMO\tFranklin County\tH1\n63080\t29071\tSullivan\tMO\tFranklin County\tH1\n63014\t29071\tBerger\tMO\tFranklin County\tH1\n63077\t29071\tSaint clair\tMO\tFranklin County\tH1\n63090\t29071\tWashington\tMO\tFranklin County\tH1\n63069\t29071\tPacific\tMO\tFranklin County\tH1\n65453\t29071\tCuba\tMO\tFranklin County\tH1\n63091\t29071\tRosebud\tMO\tFranklin County\tH1\n63073\t29071\tSaint albans\tMO\tFranklin County\tH1\n63041\t29071\tGrubville\tMO\tFranklin County\tH1\n63037\t29071\tGerald\tMO\tFranklin County\tH1\n63060\t29071\tLonedell\tMO\tFranklin County\tH1\n63013\t29071\tBeaufort\tMO\tFranklin County\tH1\n63015\t29071\tCatawissa\tMO\tFranklin County\tH1\n63072\t29071\tRobertsville\tMO\tFranklin County\tH1\n65559\t29073\tSaint james\tMO\tGasconade County\tH1\n65062\t29073\tMount sterling\tMO\tGasconade County\tH1\n63068\t29073\tNew haven\tMO\tGasconade County\tH1\n65014\t29073\tBland\tMO\tGasconade County\tH1\n63014\t29073\tBerger\tMO\tGasconade County\tH1\n65041\t29073\tHermann\tMO\tGasconade County\tH1\n65453\t29073\tCuba\tMO\tGasconade County\tH1\n63091\t29073\tRosebud\tMO\tGasconade County\tH1\n65061\t29073\tMorrison\tMO\tGasconade County\tH1\n63037\t29073\tGerald\tMO\tGasconade County\tH1\n65024\t29073\tChamois\tMO\tGasconade County\tH1\n65066\t29073\tOwensville\tMO\tGasconade County\tH1\n64441\t29075\tDenver\tMO\tGentry County\tH1\n64463\t29075\tKing city\tMO\tGentry County\tH1\n64489\t29075\tStanberry\tMO\tGentry County\tH1\n64453\t29075\tGentry\tMO\tGentry County\tH1\n64438\t29075\tDarlington\tMO\tGentry County\tH1\n64670\t29075\tPattonsburg\tMO\tGentry County\tH1\n64499\t29075\tWorth\tMO\tGentry County\tH1\n64471\t29075\tNew hampton\tMO\tGentry County\tH1\n64402\t29075\tAlbany\tMO\tGentry County\tH1\n64479\t29075\tRavenwood\tMO\tGentry County\tH1\n64657\t29075\tMc fall\tMO\tGentry County\tH1\n65890\t29077\tSpringfield\tMO\tGreene County\tH1\n65898\t29077\tSpringfield\tMO\tGreene County\tH1\n65806\t29077\tSpringfield\tMO\tGreene County\tH1\n65802\t29077\tSpringfield\tMO\tGreene County\tH1\n65706\t29077\tMarshfield\tMO\tGreene County\tH1\n65765\t29077\tTurners\tMO\tGreene County\tH1\n65803\t29077\tSpringfield\tMO\tGreene County\tH1\n65721\t29077\tOzark\tMO\tGreene County\tH1\n65725\t29077\tPleasant hope\tMO\tGreene County\tH1\n65770\t29077\tWalnut grove\tMO\tGreene County\tH1\n65610\t29077\tBillings\tMO\tGreene County\tH1\n65604\t29077\tAsh grove\tMO\tGreene County\tH1\n65804\t29077\tSpringfield\tMO\tGreene County\tH1\n65738\t29077\tRepublic\tMO\tGreene County\tH1\n65808\t29077\tSpringfield\tMO\tGreene County\tH1\n65809\t29077\tSpringfield\tMO\tGreene County\tH1\n65757\t29077\tStrafford\tMO\tGreene County\tH1\n65781\t29077\tWillard\tMO\tGreene County\tH1\n65619\t29077\tBrookline\tMO\tGreene County\tH1\n65814\t29077\tSpringfield\tMO\tGreene County\tH1\n65612\t29077\tBois d arc\tMO\tGreene County\tH1\n65807\t29077\tSpringfield\tMO\tGreene County\tH1\n65801\t29077\tSpringfield\tMO\tGreene County\tH1\n65648\t29077\tFair grove\tMO\tGreene County\tH1\n65810\t29077\tSpringfield\tMO\tGreene County\tH1\n65805\t29077\tSpringfield\tMO\tGreene County\tH1\n65617\t29077\tBrighton\tMO\tGreene County\tH1\n65742\t29077\tRogersville\tMO\tGreene County\tH1\n65897\t29077\tSpringfield\tMO\tGreene County\tH1\n65899\t29077\tSpringfield\tMO\tGreene County\tH1\n64641\t29079\tGalt\tMO\tGrundy County\tH1\n64679\t29079\tSpickard\tMO\tGrundy County\tH1\n64648\t29079\tJamesport\tMO\tGrundy County\tH1\n64635\t29079\tChula\tMO\tGrundy County\tH1\n64652\t29079\tLaredo\tMO\tGrundy County\tH1\n64642\t29079\tGilman city\tMO\tGrundy County\tH1\n64683\t29079\tTrenton\tMO\tGrundy County\tH1\n64458\t29081\tHatfield\tMO\tHarrison County\tH1\n64442\t29081\tEagleville\tMO\tHarrison County\tH1\n64426\t29081\tBlythedale\tMO\tHarrison County\tH1\n64456\t29081\tGrant city\tMO\tHarrison County\tH1\n64670\t29081\tPattonsburg\tMO\tHarrison County\tH1\n64632\t29081\tCainsville\tMO\tHarrison County\tH1\n64481\t29081\tRidgeway\tMO\tHarrison County\tH1\n64642\t29081\tGilman city\tMO\tHarrison County\tH1\n64471\t29081\tNew hampton\tMO\tHarrison County\tH1\n64424\t29081\tBethany\tMO\tHarrison County\tH1\n64467\t29081\tMartinsville\tMO\tHarrison County\tH1\n64657\t29081\tMc fall\tMO\tHarrison County\tH1\n64636\t29081\tCoffey\tMO\tHarrison County\tH1\n64740\t29083\tDeepwater\tMO\tHenry County\tH1\n64735\t29083\tClinton\tMO\tHenry County\tH1\n64724\t29083\tAppleton city\tMO\tHenry County\tH1\n64733\t29083\tChilhowee\tMO\tHenry County\tH1\n64726\t29083\tBlairstown\tMO\tHenry County\tH1\n65323\t29083\tCalhoun\tMO\tHenry County\tH1\n65360\t29083\tWindsor\tMO\tHenry County\tH1\n64770\t29083\tMontrose\tMO\tHenry County\tH1\n64788\t29083\tUrich\tMO\tHenry County\tH1\n64761\t29083\tLeeton\tMO\tHenry County\tH1\n64739\t29083\tCreighton\tMO\tHenry County\tH1\n65668\t29085\tHermitage\tMO\tHickory County\tH1\n65732\t29085\tPreston\tMO\tHickory County\tH1\n65634\t29085\tCross timbers\tMO\tHickory County\tH1\n65724\t29085\tPittsburg\tMO\tHickory County\tH1\n65779\t29085\tWheatland\tMO\tHickory County\tH1\n65774\t29085\tWeaubleau\tMO\tHickory County\tH1\n65767\t29085\tUrbana\tMO\tHickory County\tH1\n65735\t29085\tQuincy\tMO\tHickory County\tH1\n64466\t29087\tMaitland\tMO\tHolt County\tH1\n64437\t29087\tCraig\tMO\tHolt County\tH1\n64446\t29087\tFairfax\tMO\tHolt County\tH1\n64487\t29087\tSkidmore\tMO\tHolt County\tH1\n64473\t29087\tOregon\tMO\tHolt County\tH1\n64470\t29087\tMound city\tMO\tHolt County\tH1\n64451\t29087\tForest city\tMO\tHolt County\tH1\n65279\t29089\tRocheport\tMO\tHoward County\tH1\n65248\t29089\tFayette\tMO\tHoward County\tH1\n65250\t29089\tFranklin\tMO\tHoward County\tH1\n65256\t29089\tHarrisburg\tMO\tHoward County\tH1\n65281\t29089\tSalisbury\tMO\tHoward County\tH1\n65254\t29089\tGlasgow\tMO\tHoward 
